vi "Secure WebSocket Client Test.vi"() -> ()   [LabVIEW 2013]
uses:
  SSL_Lib/SSL-Lib/Library Paths.ctl
  SSL_Lib/SSL-Context/SSL Verify Mode.ctl
  SSL_Lib/SSL-Context/SSL Options.ctl
  SSL Client Context/SSL Client Context.lvclass/SSL Client Context.ctl
  SSL Client Context/SSL Client Context.lvclass
  SSL Client Socket/SSL Client Socket.lvclass
  <vilib>/MediaMongrels Ltd/WebSockets/WebSockets/WebSocket Client/WebSocket Client.lvclass
  <vilib>/MediaMongrels Ltd/WebSockets/WebSockets/WebSocket/WebSocket.lvclass/WebSocket.ctl
  SSL Client Context/Write Verification Options.vi
  SSL Client Context/Write Verification CA Bundle Path.vi
  SSL Client Context/Write SSL Options.vi
  SSL Client Context/Write Cipher List.vi
  <vilib>/MediaMongrels Ltd/WebSockets/WebSockets/WebSocket/Read Return Headers.vi
  SSL_Lib/SSL-Lib/SSL-Lib.lvclass
  SSL_Lib/SSL-Context/SSL-Context.lvclass
panel:
  out "Return Headers 2":variant
  out "Data 2":string
  out "Data":string
  out "Return Headers":variant
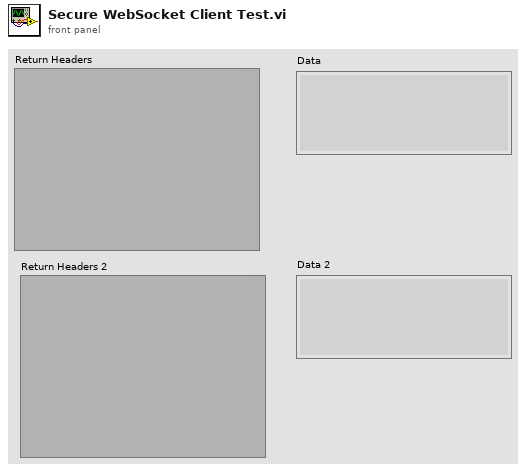
[diagram p1: front panel]
types:
  T1 = typedef "SSL_Lib.lvlib/SSL-Context.lvclass/SSL Options.ctl" = i32
  T2 = typedef "SSL_Lib.lvlib/SSL-Context.lvclass/SSL Verify Mode.ctl" = i32
  T3 = typedef "SSL_Lib.lvlib/SSL-Lib.lvclass/Library Paths.ctl" = cluster{"SSL Library Path":path, "Crypto Library Path":path}
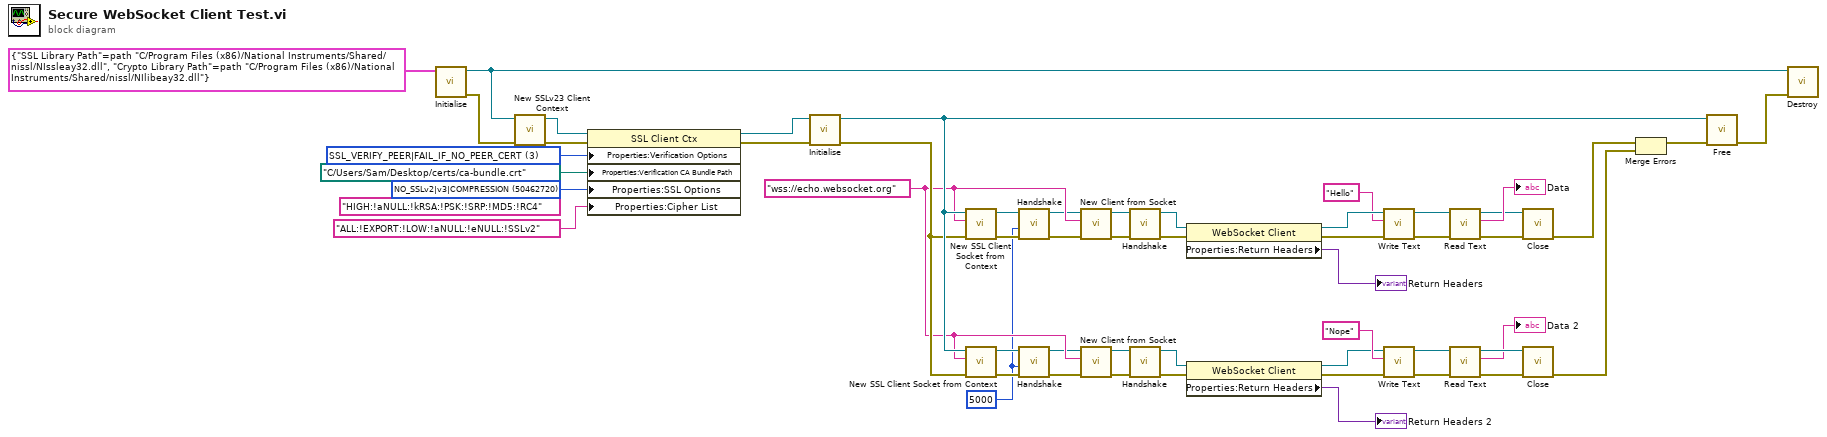
[diagram p0: block diagram]
diagram:
  w1 = u32 5000 ("Timeout (5000ms)")
  (unwired) "HIGH:!aNULL:!kRSA:!PSK:!SRP:!MD5:!RC4" ("Cipher List")
  w29 = T1 50462720 items=["None"=0, "NO_SSLv2|v3|COMPRESSION"=50462720, "SSL_OP_NO_COMPRESSION"=131072, "SSL_OP_NO_SSLv2"=16777216, "SSL_OP_NO_SSLv3"=33554432, "SSL_OP_NO_TLSv1"=67108864, "SSL_OP_NO_TLSv1_2"=134217728, "SSL_OP_NO_TLSv1_1"=268435456] ("SSL Options")
  w31 = T2 3 items=["SSL_VERIFY_PEER|FAIL_IF_NO_PEER_CERT"=3, "SSL_VERIFY_NONE"=0, "SSL_VERIFY_PEER"=1, "SSL_VERIFY_FAIL_IF_NO_PEER_CERT"=2, "SSL_VERIFY_CLIENT_ONCE"=4] ("Verification Options")
  w10 = "wss://echo.websocket.org" ("WebSocket URL")
  n1 = call "Initialise.vi"("Library Paths"=T3 {"SSL Library Path"=path "C:/Program Files (x86)/National Instruments/Shared/nissl/NIssleay32.dll", "Crypto Library Path"=path "C:/Program Files (x86)/National Instruments/Shared/nissl/NIlibeay32.dll"}) -> ("error out"=w39:errorcluster, "SSL-Lib out"=w37:refnum<class "SSL-Lib.lvclass">)  [unwired: 9 in]
  n2 = call "New SSLv23 Client Context.vi"("error in (no error)"=w39, "SSL-Lib"=w37) -> ("error out"=w38:errorcluster, "SSL Client Context out"=w33:refnum<class "SSL Client Context.lvclass">)  [unwired: 8 in]
  n3 = property class="SSL Client Ctx"(reference=w33, error in=w38, "Properties:Verification Options"=w31, "Properties:Verification CA Bundle Path"=path "C:/Users/Sam/Desktop/certs/ca-bundle.crt" ("Path to CA bundle"), "Properties:SSL Options"=w29, "Properties:Cipher List"="ALL:!EXPORT:!LOW:!aNULL:!eNULL:!SSLv2" ("Cipher List")) -> (reference out=w32:refnum<class "SSL Client Context.lvclass">, error out=w34:errorcluster)
  n4 = call-dynamic "Initialise.vi"("error in (no error)"=w34, "OpenSSL Client Context in"=w32) -> ("error out"=w11:errorcluster, "OpenSSL Client Context out"=w12:refnum<class "SSL Client Context.lvclass">)  [unwired: 8 in]
  n5 = call "New SSL Client Socket from Context.vi"("error in (no error)"=w11, "Hostname / URL"=w10, "SSL Client Ctx"=w12) -> ("error out"=w6:errorcluster, "SSL Client Skt out"=w27:refnum<class "SSL Client Socket.lvclass">)  [unwired: 7 in]
  n6 = call "New SSL Client Socket from Context.vi"("error in (no error)"=w11, "Hostname / URL"=w10, "SSL Client Ctx"=w12) -> ("error out"=w3:errorcluster, "SSL Client Skt out"=w26:refnum<class "SSL Client Socket.lvclass">)  [unwired: 7 in]
  n7 = call-dynamic "Handshake.vi"("error in (no error)"=w6, "Timeout (5000ms)"=w1, "OpenSSL in"=w27) -> ("error out"=w5:errorcluster, "OpenSSL out"=w7:refnum<class "SSL Client Socket.lvclass">)  [unwired: 7 in]
  n8 = call-dynamic "Handshake.vi"("error in (no error)"=w3, "Timeout (5000ms)"=w1, "OpenSSL in"=w26) -> ("error out"=w2:errorcluster, "OpenSSL out"=w4:refnum<class "SSL Client Socket.lvclass">)  [unwired: 7 in]
  n9 = call <vilib>:"New Client from Socket.vi"("error in (no error)"=w5, "WebSocket URL"=w10, "Socket in"=w7) -> ("error out"=w53:errorcluster, "WebSocket Client out"=w52:refnum<class "WebSocket Client.lvclass">)  [unwired: 7 in]
  n10 = call <vilib>:"New Client from Socket.vi"("error in (no error)"=w2, "WebSocket URL"=w10, "Socket in"=w4) -> ("error out"=w13:errorcluster, "WebSocket Client out"=w14:refnum<class "WebSocket Client.lvclass">)  [unwired: 7 in]
  n11 = call-dynamic "Handshake.vi"("error in (no error)"=w53, "WebSocket Client in"=w52) -> ("error out"=w51:errorcluster, "WebSocket Client out"=w50:refnum<class "WebSocket Client.lvclass">)  [unwired: 8 in]
  n12 = call-dynamic "Handshake.vi"("error in (no error)"=w13, "WebSocket Client in"=w14) -> ("error out"=w15:errorcluster, "WebSocket Client out"=w16:refnum<class "WebSocket Client.lvclass">)  [unwired: 8 in]
  n13 = property class="WebSocket Client"(reference=w50, error in=w51) -> (reference out=w47:refnum<class "WebSocket Client.lvclass">, error out=w48:errorcluster, "Properties:Return Headers"=→"Return Headers":variant)
  n14 = property class="WebSocket Client"(reference=w16, error in=w15) -> (reference out=w19:refnum<class "WebSocket Client.lvclass">, error out=w18:errorcluster, "Properties:Return Headers"=→"Return Headers 2":variant)
  n15 = call-dynamic "Write Text.vi"("error in (no error)"=w48, "String Data"="Hello", "WebSocket in"=w47) -> ("error out"=w45:errorcluster, "WebSocket out"=w44:refnum<class "WebSocket Client.lvclass">)  [unwired: 7 in]
  n16 = call-dynamic "Write Text.vi"("error in (no error)"=w18, "String Data"="Nope", "WebSocket in"=w19) -> ("error out"=w21:errorcluster, "WebSocket out"=w22:refnum<class "WebSocket Client.lvclass">)  [unwired: 7 in]
  n17 = call-dynamic "Read Text.vi"("error in (no error)"=w45, "WebSocket in"=w44) -> ("error out"=w42:errorcluster, "Data"=→"Data":string, "WebSocket out"=w41:refnum<class "WebSocket Client.lvclass">)  [unwired: 7 in]
  n18 = call-dynamic "Read Text.vi"("error in (no error)"=w21, "WebSocket in"=w22) -> ("error out"=w24:errorcluster, "Data"=→"Data 2":string, "WebSocket out"=w25:refnum<class "WebSocket Client.lvclass">)  [unwired: 7 in]
  n19 = call-dynamic "Close.vi"("error in (no error)"=w42, "WebSocket in"=w41) -> ("error out"=w35:errorcluster)  [unwired: 9 in]
  n20 = call-dynamic "Close.vi"("error in (no error)"=w24, "WebSocket in"=w25) -> ("error out"=w8:errorcluster)  [unwired: 9 in]
  n21 = Merge Errors(w35, w8) -> (w9:errorcluster)
  n22 = call-dynamic "Free.vi"("error in (no error)"=w9, "OpenSSL Context in"=w12) -> ("error out"=w36:errorcluster)  [unwired: 9 in]
  n23 = call "Destroy.vi"("error in (no error)"=w36, "SSL-Lib in"=w37) -> ()  [unwired: 9 in, 1 out]
